vi "mupExpr Plot.vi"() -> ()   [LabVIEW 2015]
uses:
  <vilib>/Utility/error.llb/DialogType.ctl
  mupExpr/mupExpr.lvclass/mupExpr.ctl
  mupExpr/Eval_SglVar_BulkMode.vi
  mupLib/mupEvalBulk.vi
  mupLib/mupSetVarValue_Array.vi
  mupLib/mupCheckError.vi
  mupLib/mupLibPath.vi
  <vilib>/Utility/error.llb/Error Cluster From Error Code.vi
  mupExpr/mupExpr.lvclass
panel:
  in  "Expression":string="sin(x)"
  in  "Increment":dbl=0.01
  in  "Start":dbl
  in  "End":dbl=6.283
  in  "Plot":bool
  out "XY Graph":cluster{dbl[], "Result":dbl[]}(graph)
  # "Single Variable \"x\""
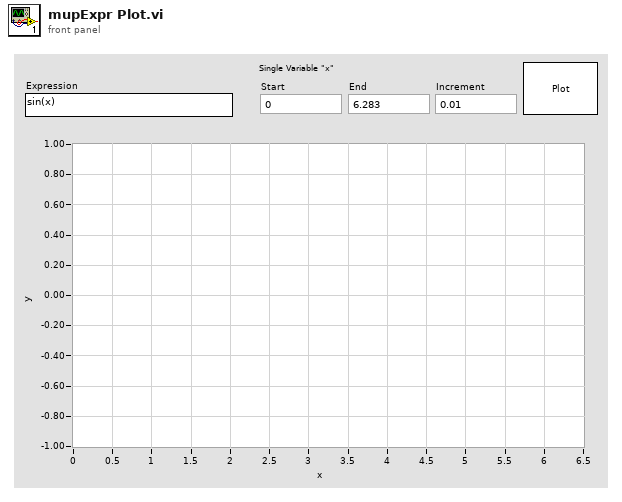
[diagram p1: front panel]
types:
  T1 = typedef "DialogType.ctl" = u16
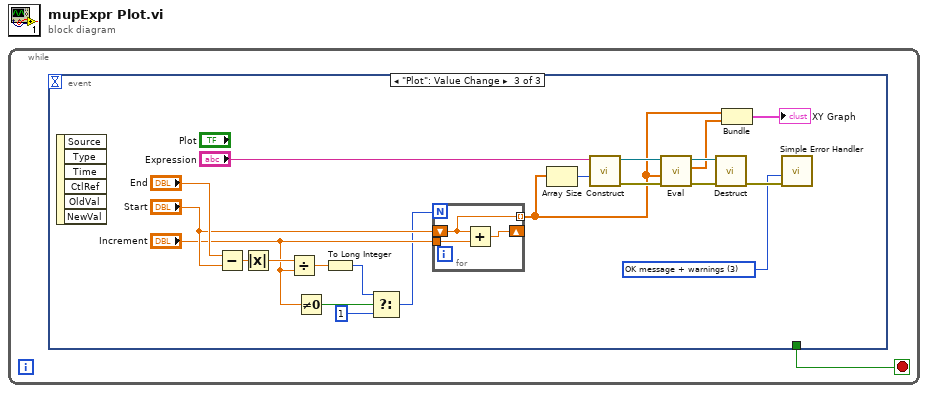
[diagram p0: block diagram]
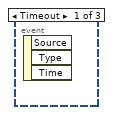
[diagram p2: hidden frame]
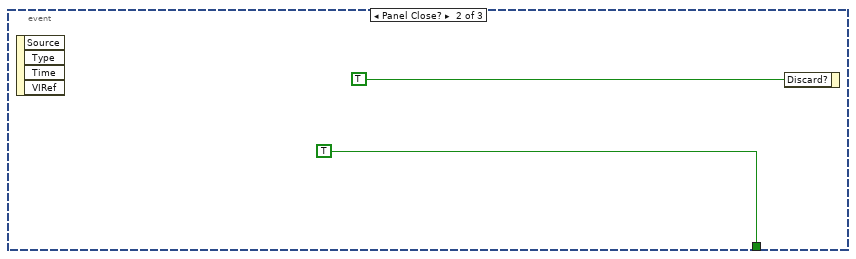
[diagram p3: hidden frame]
diagram:
  n1 = while {
    stop <- w1 stop-if-true
    n2 = event shown="[2] \"Plot\": Value Change" {
      selector: _ -> [_ _ _]
      dyn-events: _ -> [_ _ _]
      timeout: _ -> [_ _ _]
      tunnel: [_ TRUE _] -> w1
      event Timeout {
        n3 = event-data() -> ()  [unwired: 1 in, 3 out]
      }
      event Panel Close? {
        n4 = event-data() -> ()  [unwired: 1 in, 4 out]
        n5 = event-data("Discard?"=TRUE) -> ()  [unwired: 1 in, 1 out]
      }
      event "Plot": Value Change {
        w9 = T1 3 items=["no dialog", "OK message", "continue or stop message", "OK message + warnings", "continue/stop + warnings"] ("type of dialog (OK msg:1)")
        n6 = event-data() -> ()  [unwired: 1 in, 6 out]
        n7 = Subtract(x="End", y="Start") -> (x-y=w21:dbl)
        n8 = Absolute Value(x=w21) -> (abs(x)=w22:dbl)
        n9 = Divide(x=w22, y="Increment") -> (x/y=w23:dbl)
        n10 = Not Equal To 0?(x="Increment") -> (x != 0?=w20:bool)
        n11 = To Long Integer(number=w23) -> (32bit integer=w19:i32)
        n12 = Select(t=w19, s=w20, f=1) -> (s? t:f=w6:i32)
        n13 = for {
          N: w6 -> [_]
          tunnel: "Increment" -> [w27]
          shift-right: [w26] -> _
          shift-left: "Start" -> [w25]
          tunnel: [w25] -> w5 mode=indexing
          n14 = Add(x=w25, y=w27) -> (x+y=w26:dbl)
        }
        n15 = Array Size(array=w5) -> (size(s)=w4:i32)
        n16 = call "Construct.vi"("Bulk Size (1)"=w4, "Expression"="Expression") -> ("error out"=w13:errorcluster, "mupExpr out"=w14:refnum<data-value>)  [unwired: 7 in, 1 out]
        n17 = call-poly "Eval.vi"("error in (no error)"=w13, "varValue"=w5, "mupExpr in"=w14) -> ("error out"=w11:errorcluster, "Result"=w8:dbl[], "mupExpr out"=w12:refnum<data-value>)  [unwired: 6 in]
        n18 = call "Destruct.vi"("error in (no error)"=w11, "mupExpr in"=w12) -> ("error out"=w10:errorcluster)  [unwired: 9 in]
        n19 = Bundle(w5, "Result"=w8) -> (→"XY Graph":cluster{dbl[], "Result":dbl[]})  [unwired: 1 in]
        n20 = call <vilib>:"Simple Error Handler.vi"("type of dialog (OK msg:1)"=w9, "error in (no error)"=w10) -> ()  [unwired: 3 in, 5 out]
      }
    }
  }
